vi "_readBufferNames.vi"(11 "Data Value Reference in":refnum<data-value>) -> (2 "Names":string[](array[string]), 3 "Data Value Reference out":refnum<data-value>)   [LabVIEW 2013, in "CircularBuffer.lvlib" / "VariantBufferMap.lvclass"]
uses:
  VariantBufferMap.lvclass
  VariantBuffer/VariantBuffer.lvclass
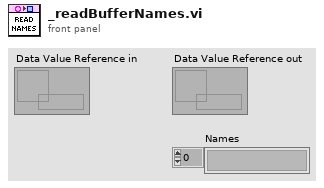
[diagram p1: front panel]
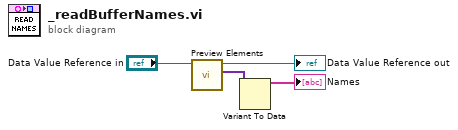
[diagram p0: block diagram]
diagram:
  n1 = call "Preview Elements.vi"("ByteBuffer in"="Data Value Reference in") -> ("elements"=w2:variant[], "ByteBuffer"=→"Data Value Reference out":refnum<data-value>)  [unwired: 8 in, 1 out]
  n2 = Variant To Data(Variant=w2) -> (data=→"Names":string[])  [unwired: 2 in, 1 out]
